vi "Test TTL Expression Edit.vi"() -> ()   [LabVIEW 2015]
uses:
  Typedefs/TTLController XControl/TTLController.xctl
  Control Classes/Base Class/TTLController.lvclass
panel:
  in  "stop":bool
  in  "TTLController":refnum<class "TTLController.lvclass">(xcontrol)
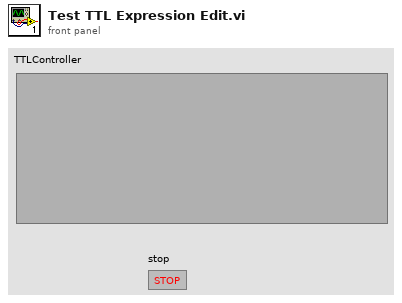
[diagram p1: front panel]
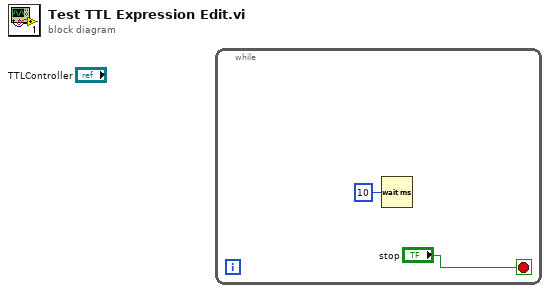
[diagram p0: block diagram]
diagram:
  n1 = while {
    stop <- "stop" stop-if-true
    n2 = Wait (ms)(milliseconds to wait=u32 10) -> ()  [unwired: 1 out]
  }
